vi "CompoundWaveformGen.vi"(0 "Fundamental Frequency":dbl, 1 "Third Harmonic":T1(ring), 5 "A third":T1(ring), 7 "A second":T1(ring), 9 "Fundamental":T1(ring), 11 "Second Harmonic":T1(ring)) -> (4 "signal out":waveform(dbl))   [LabVIEW 2016]
uses:
  <vilib>/measure/NI_MABase.lvlib
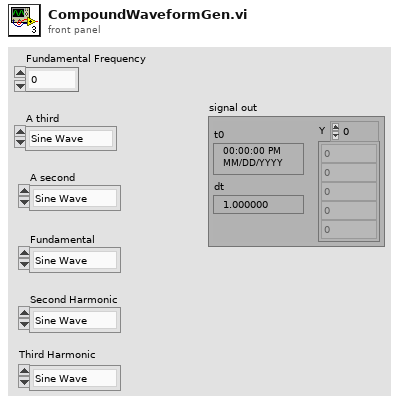
[diagram p1: front panel]
types:
  T1 = enum16{"Sine Wave", "Triangle Wave", "Square Wave", "Sawtooth Wave"}
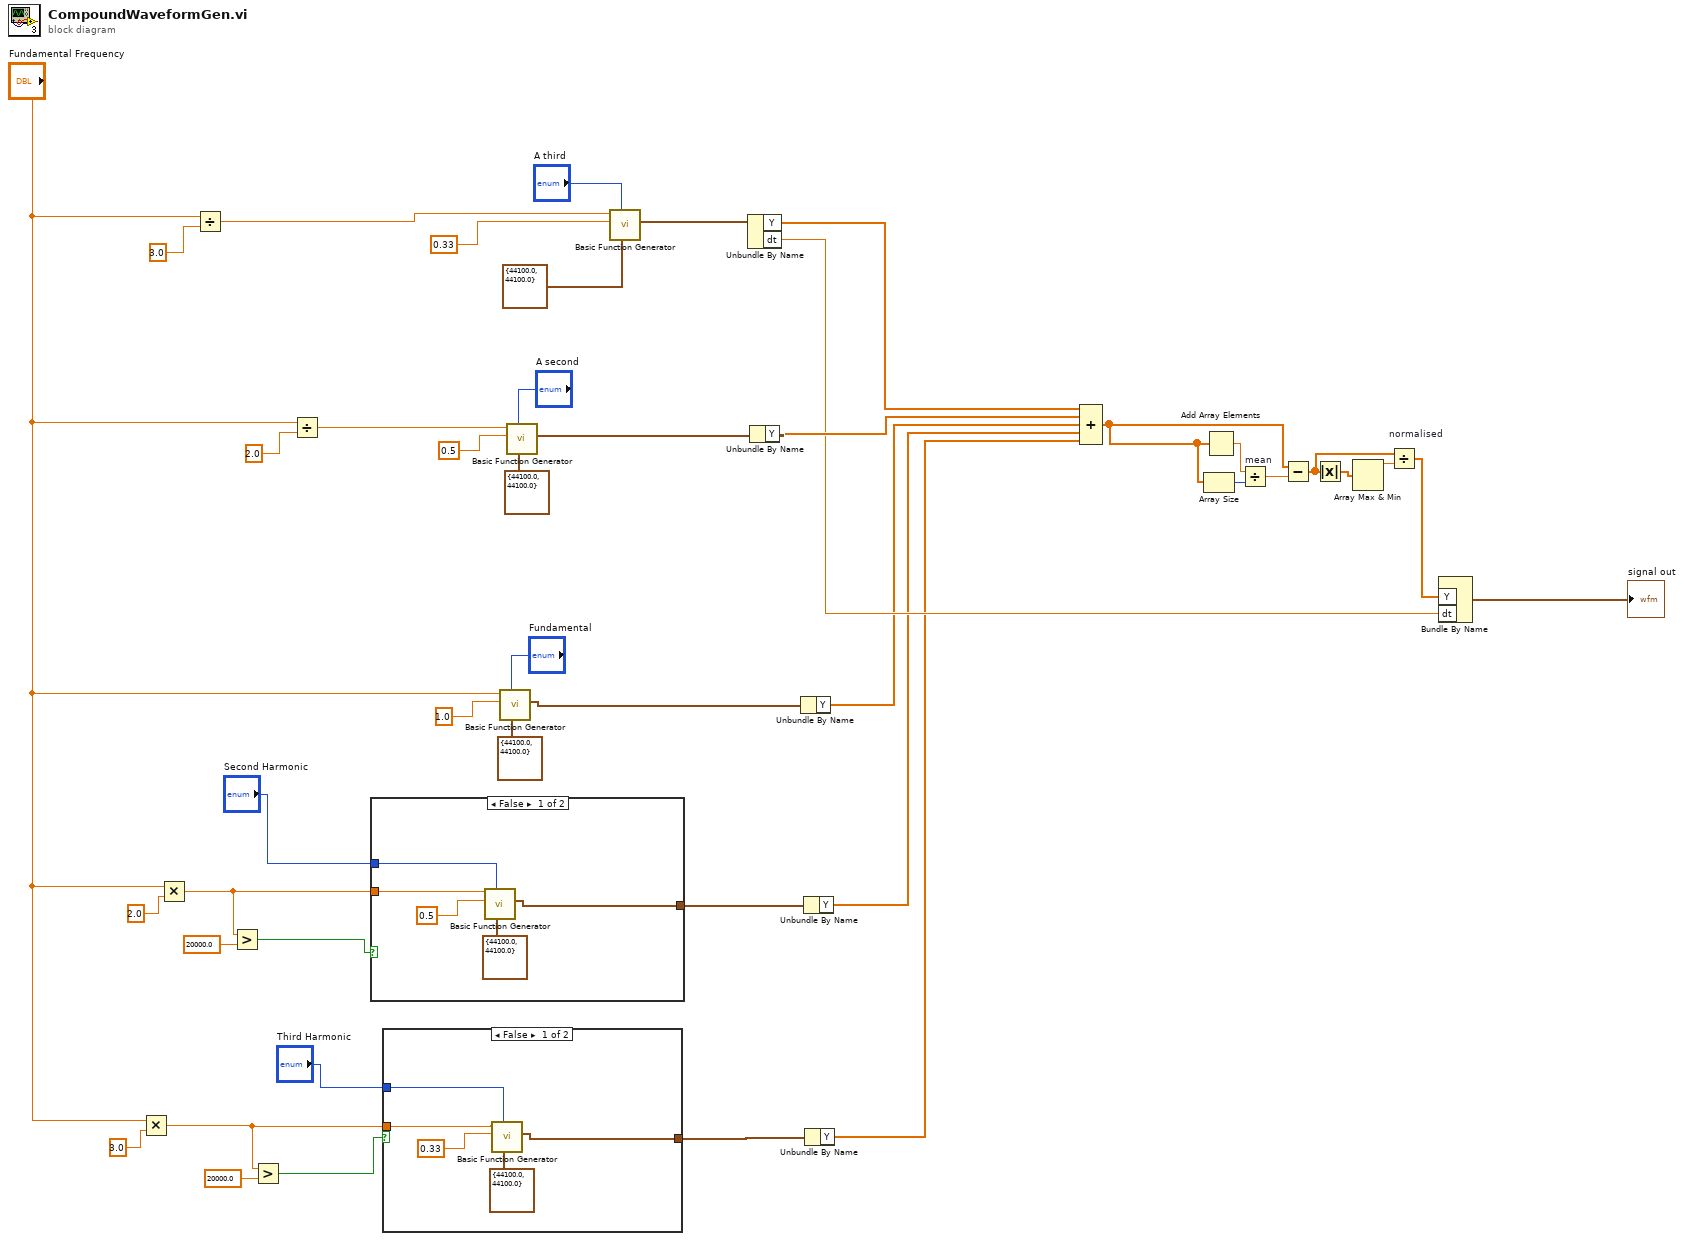
[diagram p0: block diagram]
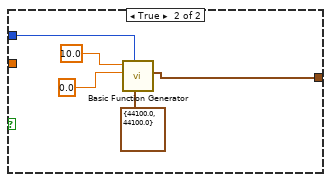
[diagram p2: hidden frame]
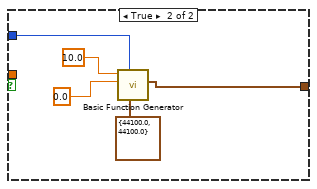
[diagram p3: hidden frame]
diagram:
  n1 = Multiply(x="Fundamental Frequency", y=3.0) -> (x*y=w16:dbl)
  n2 = Multiply(x="Fundamental Frequency", y=2.0) -> (x*y=w12:dbl)
  n3 = Divide(x="Fundamental Frequency", y=3.0) -> (x/y=w41:dbl)
  n4 = Greater?(x=w12, y=20000.0) -> (0:w11:bool)
  n5 = Greater?(x=w16, y=20000.0) -> (0:w14:bool)
  n6 = Divide(x="Fundamental Frequency", y=2.0) -> (x/y=w17:dbl)
  n7 = case shown="False" w11 {
    tunnel: [w47 w52] -> w25
    tunnel: w12 -> [w46 _]
    tunnel: "Second Harmonic" -> [w45 w51]
    frame False {
      n8 = call <vilib>:"Basic Function Generator.vi"("sampling info"=cluster{"Fs":dbl, "#s":dbl} {"Fs"=44100.0, "#s"=44100.0}, "signal type"=w45, "amplitude"=0.5, "frequency"=w46) -> ("signal out"=w47:waveform(dbl))  [unwired: 5 in, 2 out]
    }
    frame True {
      n9 = call <vilib>:"Basic Function Generator.vi"("sampling info"=cluster{"Fs":dbl, "#s":dbl} {"Fs"=44100.0, "#s"=44100.0}, "signal type"=w51, "amplitude"=0.0, "frequency"=10.0) -> ("signal out"=w52:waveform(dbl))  [unwired: 5 in, 2 out]
    }
  }
  n10 = case shown="False" w14 {
    tunnel: [w57 w62] -> w23
    tunnel: w16 -> [w56 _]
    tunnel: "Third Harmonic" -> [w55 w61]
    frame False {
      n11 = call <vilib>:"Basic Function Generator.vi"("sampling info"=cluster{"Fs":dbl, "#s":dbl} {"Fs"=44100.0, "#s"=44100.0}, "signal type"=w55, "amplitude"=0.33, "frequency"=w56) -> ("signal out"=w57:waveform(dbl))  [unwired: 5 in, 2 out]
    }
    frame True {
      n12 = call <vilib>:"Basic Function Generator.vi"("sampling info"=cluster{"Fs":dbl, "#s":dbl} {"Fs"=44100.0, "#s"=44100.0}, "signal type"=w61, "amplitude"=0.0, "frequency"=10.0) -> ("signal out"=w62:waveform(dbl))  [unwired: 5 in, 2 out]
    }
  }
  n13 = call <vilib>:"Basic Function Generator.vi"("sampling info"=cluster{"Fs":dbl, "#s":dbl} {"Fs"=44100.0, "#s"=44100.0}, "signal type"="Fundamental", "amplitude"=1.0, "frequency"="Fundamental Frequency") -> ("signal out"=w24:waveform(dbl))  [unwired: 5 in, 2 out]
  n14 = call <vilib>:"Basic Function Generator.vi"("sampling info"=cluster{"Fs":dbl, "#s":dbl} {"Fs"=44100.0, "#s"=44100.0}, "signal type"="A second", "amplitude"=0.5, "frequency"=w17) -> ("signal out"=w37:waveform(dbl))  [unwired: 5 in, 2 out]
  n15 = call <vilib>:"Basic Function Generator.vi"("sampling info"=cluster{"Fs":dbl, "#s":dbl} {"Fs"=44100.0, "#s"=44100.0}, "signal type"="A third", "amplitude"=0.33, "frequency"=w41) -> ("signal out"=w39:waveform(dbl))  [unwired: 5 in, 2 out]
  n16 = Unbundle By Name(w39) -> ("Y"=w38:dbl[], "dt"=w35:dbl)
  n17 = Unbundle By Name(w37) -> ("Y"=w36:dbl[])
  n18 = Unbundle By Name(w24) -> ("Y"=w34:dbl[])
  n19 = Unbundle By Name(w25) -> ("Y"=w33:dbl[])
  n20 = Unbundle By Name(w23) -> ("Y"=w32:dbl[])
  n21 = Compound Arithmetic op=ADD(w38, w36, w34, w33, w32) -> (w4:dbl[])
  n22 = Array Size(array=w4) -> (size(s)=w5:i32)
  n23 = Add Array Elements(numeric array=w4) -> (sum=w6:dbl)
  n24 = Divide "mean"(x=w6, y=w5) -> (x/y=w3:dbl)
  n25 = Subtract(x=w4, y=w3) -> (x-y=w2:dbl[])
  n26 = Absolute Value(x=w2) -> (abs(x)=w7:dbl[])
  n27 = Array Max & Min(array=w7) -> (max value=w8:dbl)  [unwired: 3 out]
  n28 = Divide "normalised"(x=w2, y=w8) -> (x/y=w1:dbl[])
  n29 = Bundle By Name("Y"=w1, "dt"=w35) -> (→"signal out":waveform(dbl))  [unwired: 1 in]
